vi "json Clone - string path.vi"(8 "error in (no error)":errorcluster, 10 "path":string, 11 "JSON Document in":refnum<class "JSON Document.lvclass">) -> (0 "error out":errorcluster, 1 "JSON Document out":refnum<class "JSON Document.lvclass">, 3 "JSON Document out":refnum<class "JSON Document.lvclass">)   [LabVIEW 2015, in "JSON Document.lvclass"]
uses:
  JSON Document.lvclass
  JSON Document.lvclass/JSON Document.ctl
  rapidjson wrapper/rapidjson wrapper.lvlib
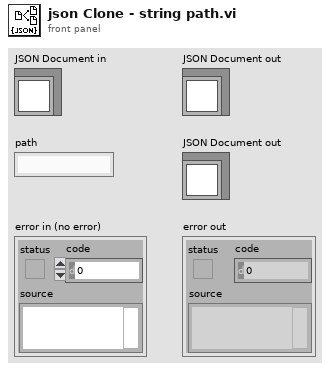
[diagram p1: front panel]
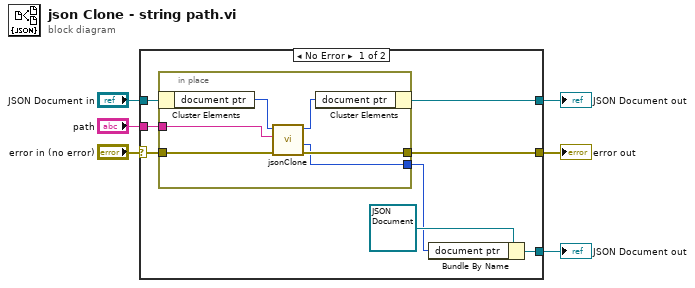
[diagram p0: block diagram]
diagram:
  n1 = case shown="No Error" "error in (no error)" {
    selector: "error in (no error)" -> [w13 w22]
    tunnel: [w12 w22] -> w5
    tunnel: [w14 w21] -> w3
    tunnel: "JSON Document in" -> [w7 w21]
    tunnel: "path" -> [w11 _]
    tunnel: [w8 _] -> w1
    frame No Error {
      n2 = in-place {
        in-place-border: w13 -> [w18]
        in-place-border: [w17] -> w12
        in-place-border: w11 -> [w16]
        in-place-border: [w15] -> w9
        n3 = in-place-cluster #1(w7) -> ("document ptr"=w20:i64)
        n4 = call "jsonClone.vi"("error in (no error)"=w18, "path"=w16, "d in"=w20) -> ("error out"=w17:errorcluster, "clone of d"=w15:i64, "d out"=w19:i64)  [unwired: 6 in]
        n5 = in-place-cluster #1("document ptr"=w19) -> (w14:refnum<class "JSON Document.lvclass">)
      }
      n6 = Bundle By Name(cluster=refnum<class "JSON Document.lvclass"> refnum ("JSON Document.lvclass"), "document ptr"=w9) -> (w8:refnum<class "JSON Document.lvclass">)
    }
    frame Error {
    }
  }
  "error out" <- w5
  "JSON Document out" <- w3
  "JSON Document out" <- w1
